vi "FilterAndAverage.vi"(11 "FilteredVisionData":T1) -> (2 "?":dbl(graph))   [LabVIEW 2018, in "Vision.lvlib" / "Vision.lvclass"]
uses:
  Vision.lvclass
  FilteredVisionData.ctl
  Controls/FGVEnum.ctl
panel:
  in  "VisionData":dbl
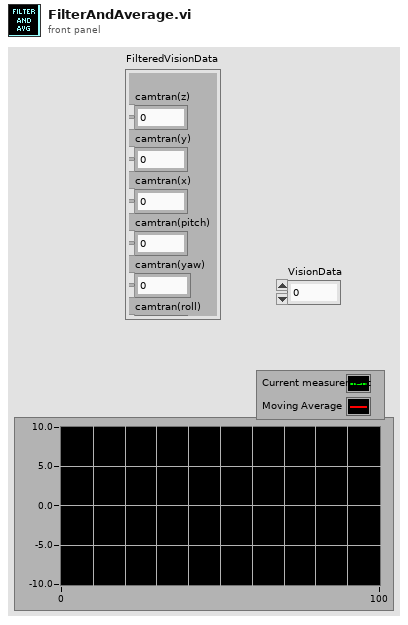
[diagram p1: front panel]
types:
  T1 = typedef "Vision.lvlib/Vision.lvclass/FilteredVisionData.ctl" = cluster{"camtran(z)":dbl, "camtran(x)":dbl, "camtran(pitch)":dbl, "camtran(y)":dbl, "camtran(roll)":dbl, "camtran(yaw)":dbl}
  T2 = typedef "Vision.lvlib/Vision.lvclass/FGVEnum.ctl" = enum16{"Read", "Write"}
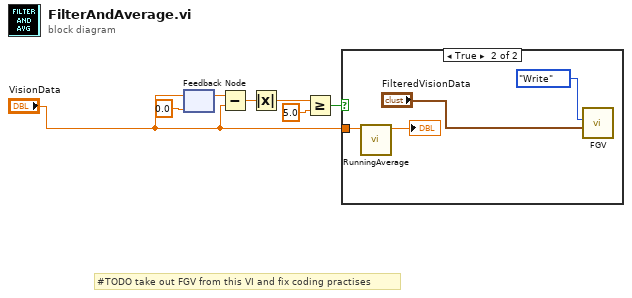
[diagram p0: block diagram]
diagram:
  # "#TODO take out FGV from this VI and fix coding practises"
  n1 = feedback #1(0.0 ("camtran (z)")) -> (w2:dbl)
  n2 = feedback-in #1("VisionData") -> ()
  n3 = Subtract(x=w2, y="VisionData") -> (x-y=w4:dbl)
  n4 = Absolute Value(x=w4) -> (abs(x)=w5:dbl)
  n5 = Greater Or Equal?(x=w5, y=5.0) -> (x >= y?=w7:bool)
  n6 = case shown="True" w7 {
    tunnel: "VisionData" -> [_ w11]
    frame False {
    }
    frame True {
      n7 = call "RunningAverage.vi"("camtran (z)"=w11) -> ("mean"=→"?":dbl)  [unwired: 10 in]
      n8 = call "FGV.vi"("FilteredVisionData"="FilteredVisionData", 10:FGVEnum."Write") -> ()  [unwired: 9 in, 1 out]
    }
  }
